vi "getHardwareList.vi"(8 "error in (no error)":errorcluster, 10 "Enum":T1(ring), 11 "HWConfiguration in":refnum<class "HWConfiguration.lvclass">) -> (0 "error out":errorcluster, 2 "HWList":string[](array[string]), 3 "HWConfiguration out":refnum<class "HWConfiguration.lvclass">)   [LabVIEW 2011, in "Hardware.lvlib" / "HWControllers.lvlib" / "HWConfiguration.lvclass"]
uses:
  HWConfiguration.lvclass
  HWConfiguration.lvclass/HWConfiguration.ctl
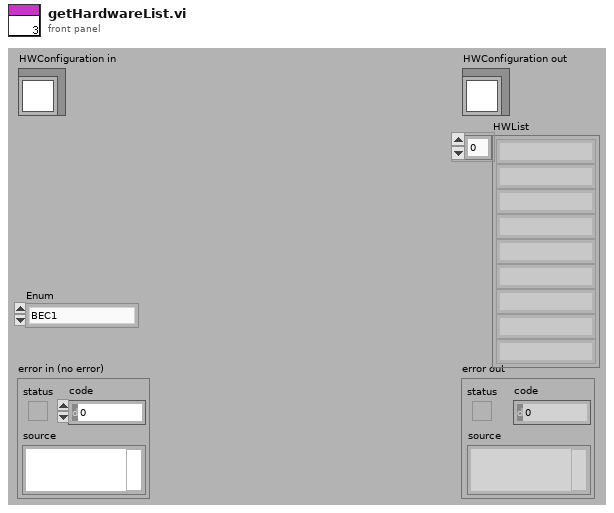
[diagram p1: front panel]
types:
  T1 = enum16{"BEC1", "BEC2", "SingleAtom", "Testing", "AtomChip"}
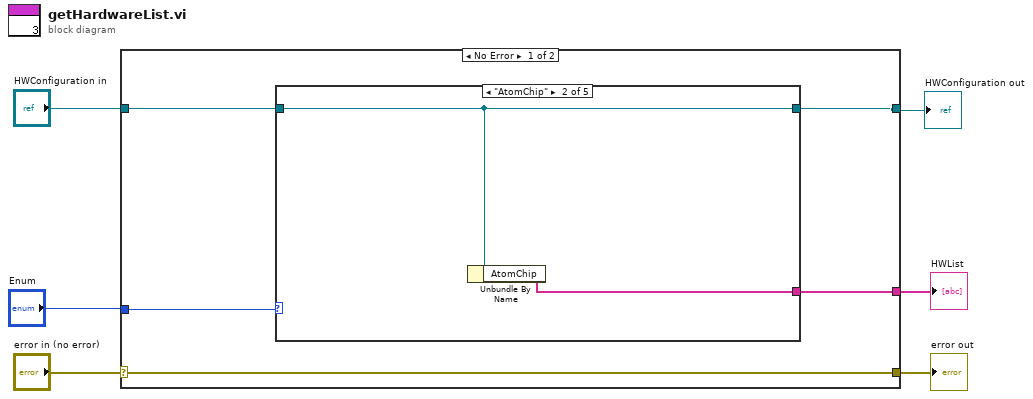
[diagram p0: block diagram]
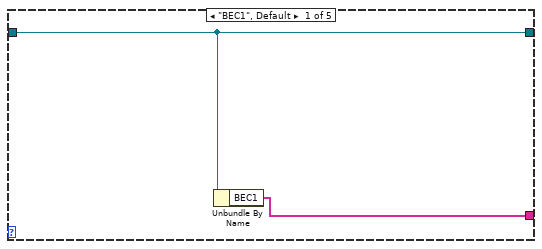
[diagram p2: hidden frame]
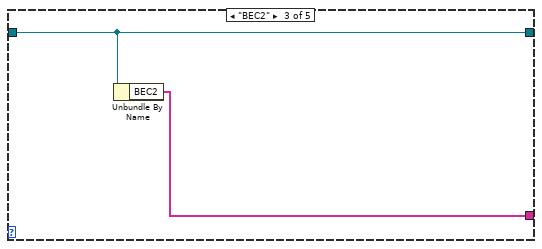
[diagram p3: hidden frame]
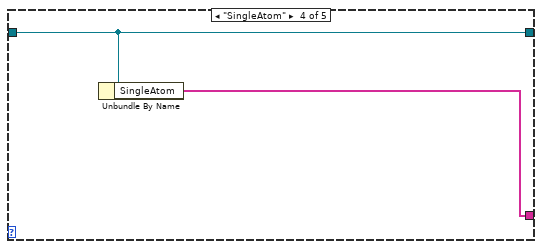
[diagram p4: hidden frame]
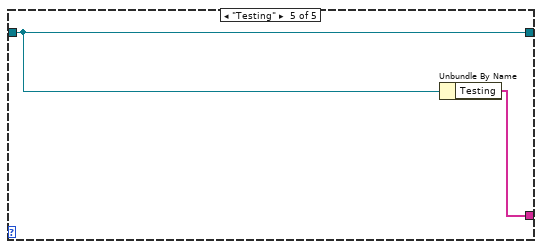
[diagram p5: hidden frame]
diagram:
  n1 = case shown="No Error" "error in (no error)" {
    selector: "error in (no error)" -> [w8 w23]
    tunnel: [w8 w23] -> w5
    tunnel: [w9 w22] -> w3
    tunnel: "HWConfiguration in" -> [w10 w22]
    tunnel: "Enum" -> [w11 _]
    tunnel: [w7 _] -> w1
    frame No Error {
      n2 = case shown="\"AtomChip\"" w11 {
        tunnel: w10 -> [w13 w15 w17 w19 w21]
        tunnel: [w13 w15 w17 w19 w21] -> w9
        tunnel: [w12 w14 w16 w18 w20] -> w7
        frame "BEC1", Default {
          n3 = Unbundle By Name(w13) -> ("BEC1"=w12:string[])
        }
        frame "AtomChip" {
          n4 = Unbundle By Name(w15) -> ("AtomChip"=w14:string[])
        }
        frame "BEC2" {
          n5 = Unbundle By Name(w17) -> ("BEC2"=w16:string[])
        }
        frame "SingleAtom" {
          n6 = Unbundle By Name(w19) -> ("SingleAtom"=w18:string[])
        }
        frame "Testing" {
          n7 = Unbundle By Name(w21) -> ("Testing"=w20:string[])
        }
      }
    }
    frame Error {
    }
  }
  "error out" <- w5
  "HWConfiguration out" <- w3
  "HWList" <- w1
